vi "InputOutputControlByIdentifier.vi"(5 "LogSuspend":bool, 8 "error in":errorcluster, 9 "ControlOption":string="02 02", 10 "DID":string="0x02 0x02", 11 "UdsHandleIn":T1={"LogPath"=path "", "LogEnabled"=FALSE, "isOpen"=FALSE, "LogContent"="", "Adapter"="CAN0", "MCanHandle"={"MCanAdapter"=refnum}, "TransmittId"=0, "ReceiveId"=0}) -> (0 "error out":errorcluster, 3 "UdsHandleOut":T1={"LogPath"=path "", "LogEnabled"=FALSE, "isOpen"=FALSE, "LogContent"="", "Adapter"="CAN0", "MCanHandle"={"MCanAdapter"=refnum}, "TransmittId"=0, "ReceiveId"=0})   [LabVIEW 2011, in "Konvolucio MUDS150628.lvlib"]
uses:
  <instrlib>/Konvolucio MUDS150628/Konvolucio MUDS150628.lvlib
  <instrlib>/Konvolucio MUDS150628/Types/UdsHandleType.ctl
  <instrlib>/Konvolucio MCAN120803/Types/MCanHandleType.ctl
  C:/Program Files/National Instruments/LabVIEW 2011/instr.lib/Konvolucio MCAN120803/Private/Konvolucio.MCAN120803.dll
  Konvolucio MCAN120803/Private/Konvolucio.MCAN120803.dll
  <instrlib>/Konvolucio MCAN120803/Konvolucio MCAN120803.lvlib
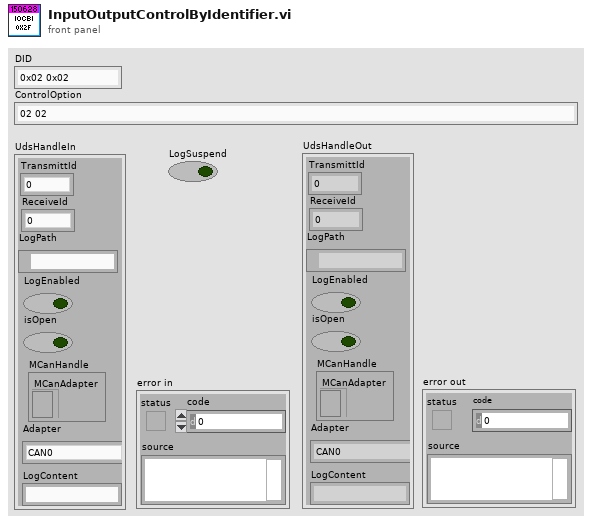
[diagram p1: front panel]
types:
  T1 = typedef "Konvolucio MUDS150628.lvlib/UdsHandleType.ctl" = cluster{"LogPath":path, "LogEnabled":bool, "isOpen":bool, "LogContent":string, "Adapter":string, "MCanHandle":T2, "TransmittId":u32, "ReceiveId":u32}
  T2 = typedef "Konvolucio MCAN120803.lvlib/MCanHandleType.ctl" = cluster{"MCanAdapter":refnum<k24>}
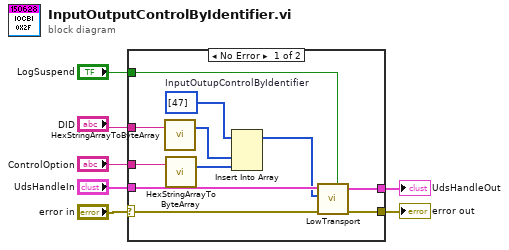
[diagram p0: block diagram]
diagram:
  n1 = case shown="No Error" "error in" {
    selector: "error in" -> [w17 w20]
    tunnel: "UdsHandleIn" -> [w18 w19]
    tunnel: [w16 w20] -> w5
    tunnel: [w15 w19] -> w4
    tunnel: "LogSuspend" -> [w14 _]
    tunnel: "DID" -> [w11 _]
    tunnel: "ControlOption" -> [w9 _]
    frame No Error {
      w13 = u8[] [47]  # InputOutupControlByIdentifier
      n2 = call <instrlib>:"HexStringArrayToByteArray.vi"("HexStirngArray"=w11) -> ("ByteArrayOut"=w10:u8[])  [unwired: 2 in]
      n3 = call <instrlib>:"HexStringArrayToByteArray.vi"("HexStirngArray"=w9) -> ("ByteArrayOut"=w8:u8[])  [unwired: 2 in]
      n4 = Insert Into Array(array=w13, new element #1=w10, new element #2=w8) -> (w12:u8[])  [unwired: 1 in]
      n5 = call <instrlib>:"LowTransport.vi"("LogSuspend"=w14, "error in"=w17, "Request"=w12, "HandleIn"=w18) -> ("error out"=w16:errorcluster, "HandleOut"=w15:T1)  [unwired: 5 in, 1 out]
    }
    frame Error {
    }
  }
  "error out" <- w5
  "UdsHandleOut" <- w4
